vi "Demarcate.vi"(7 "Mode":enum16{"Read", "Write"}(ring)=enum."Write", 8 "error in":errorcluster, 10 "工位二扭矩偏移":cluster{"正向":dbl, "逆向":dbl}, 11 "工位一扭矩偏移":cluster{"正向":dbl, "逆向":dbl}) -> (0 "error out":errorcluster, 2 "工位二扭矩偏移O":cluster{"正向":dbl, "逆向":dbl}, 3 "工位一扭矩偏移O":cluster{"正向":dbl, "逆向":dbl})   [LabVIEW 2020]
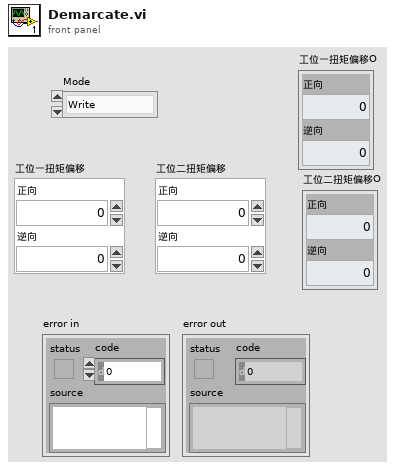
[diagram p1: front panel]
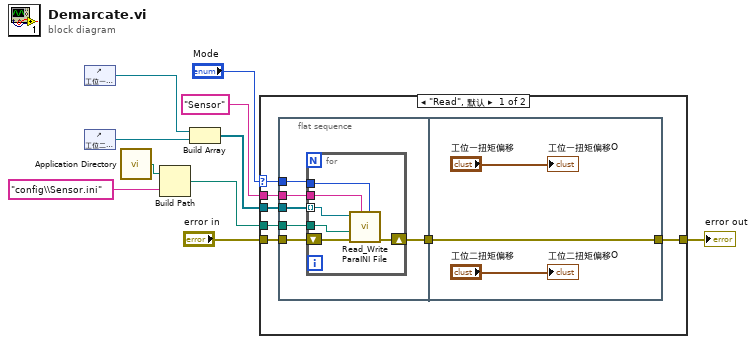
[diagram p0: block diagram]
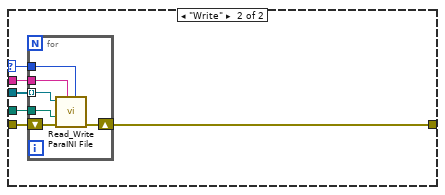
[diagram p2: hidden frame]
diagram:
  n1 = control-ref of="工位一扭矩偏移"() -> (w2:refnum<vi>)
  n2 = control-ref of="工位二扭矩偏移"() -> (w1:refnum<vi>)
  n3 = call <vilib>:"Application Directory.vi"() -> ("Application Directory"=w9:path)
  n4 = Build Path(base path=w9, name or relative path="config\\Sensor.ini" ("名称或相对路径")) -> (appended path=w7:path)
  n5 = Build Array(w2, w1) -> (w3:refnum<vi>[])
  n6 = case shown="\"Read\", 默认" "Mode" {
    selector: "Mode" -> [w15 w35]
    tunnel: w3 -> [w16 w38]
    tunnel: "Sensor" ("Section") -> [w14 w37]
    tunnel: w7 -> [w17 w36]
    tunnel: "error in" -> [w13 w34]
    tunnel: [w12 w33] -> w4
    frame "Read", Default {
      n7 = flat-sequence {
        tunnel: w17 -> [w23]
        tunnel: w16 -> [w22]
        tunnel: w15 -> [w21]
        tunnel: w14 -> [w20]
        tunnel: w13 -> [w19]
        tunnel: [w18] -> w11
        tunnel: [w32] -> w12
        tunnel: w11 -> [w32]
        frame #0 {
          n8 = for {
            tunnel: w23 -> [w29]
            tunnel: w22 -> [w28] mode=indexing
            tunnel: w21 -> [w27]
            tunnel: w20 -> [w26]
            shift-right: [w24] -> w18
            shift-left: w19 -> [w25]
            n9 = call "Read_Write ParaINI File.vi"("Mode"=w27, "Section"=w26, "error in"=w25, "Filepath"=w29, "Ctl Refnum"=w28) -> ("error out"=w24:errorcluster)  [unwired: 6 in]
          }
        }
        frame #1 {
          "工位一扭矩偏移O" <- "工位一扭矩偏移"
          "工位二扭矩偏移O" <- "工位二扭矩偏移"
        }
      }
    }
    frame "Write" {
      n10 = for {
        tunnel: w38 -> [w44] mode=indexing
        tunnel: w37 -> [w43]
        tunnel: w36 -> [w42]
        tunnel: w35 -> [w41]
        shift-right: [w39] -> w33
        shift-left: w34 -> [w40]
        n11 = call "Read_Write ParaINI File.vi"("Mode"=w41, "Section"=w43, "error in"=w40, "Filepath"=w42, "Ctl Refnum"=w44) -> ("error out"=w39:errorcluster)  [unwired: 6 in]
      }
    }
  }
  "error out" <- w4
